vi "Apply Filter_2D.vi"(6 "filter index":i32, 10 "Filter":string, 11 "Item names":string[][](array[string])) -> (3 "Filtered Item Names":string[][](array[string]))   [LabVIEW 2013, in "CVT editor node.lvclass"]
uses:
  CVT editor node.lvclass
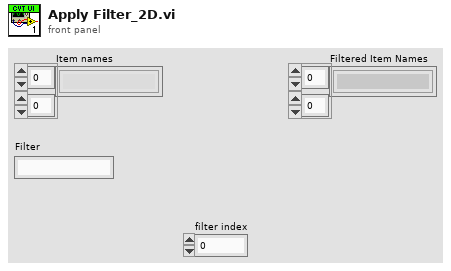
[diagram p1: front panel]
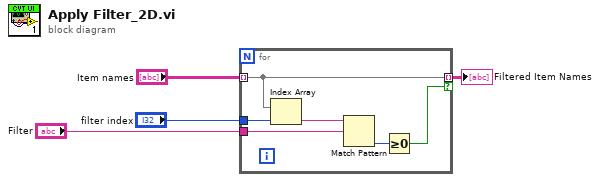
[diagram p0: block diagram]
diagram:
  n1 = for {
    tunnel: "Item names" -> [w7] mode=indexing
    tunnel: "Filter" -> [w10]
    tunnel: [w7] -> w2 mode=indexing if=w8
    tunnel: "filter index" -> [w5]
    n2 = Index Array(array=w7, index=w5) -> (element=w6:string)
    n3 = Match Pattern(string=w6, regular expression=w10) -> (offset past match=w9:i32)  [unwired: 1 in, 3 out]
    n4 = Greater Or Equal To 0?(x=w9) -> (x >= 0?=w8:bool)
  }
  "Filtered Item Names" <- w2
